vi "DAQ.DAQmx Replace Existing Task.vi"(9 "Task in":refnum<k21>, 10 "Task Index":i32, 11 "Tasks in":refnum<k21>[](array[refnum])) -> (3 "Tasks out":refnum<k21>[](array[refnum]))   [LabVIEW 2019, in "Instrument.Lockin.lvlib" / "Instrument.DAQ.lvclass"]
uses:
  Instrument.DAQ.lvclass
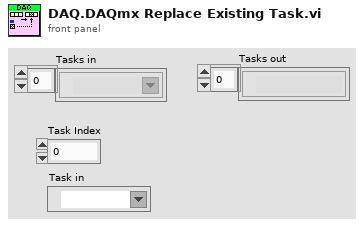
[diagram p1: front panel]
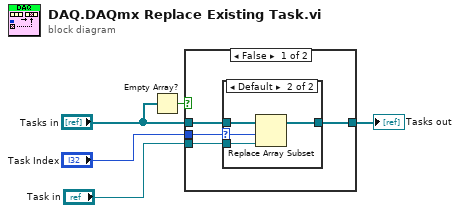
[diagram p0: block diagram]
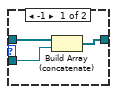
[diagram p2: hidden frame]
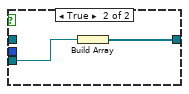
[diagram p3: hidden frame]
diagram:
  n1 = Empty Array?(array="Tasks in") -> (empty?=w1:bool)
  n2 = case shown="False" w1 {
    tunnel: [w9 w18] -> w3
    tunnel: "Task in" -> [w8 w17]
    tunnel: "Task Index" -> [w7 _]
    tunnel: "Tasks in" -> [w6 _]
    frame False {
      n3 = case shown="Default" w7 {
        selector: w7 -> [_ w14]
        tunnel: [w10 w16] -> w9
        tunnel: w8 -> [w11 w15]
        tunnel: w6 -> [w12 w13]
        frame -1 {
          n4 = Build Array (concatenate)(w12, w11) -> (w10:refnum<k21>[])
        }
        frame Default {
          n5 = Replace Array Subset(array=w13, new element=w15, index=w14) -> (w16:refnum<k21>[])
        }
      }
    }
    frame True {
      n6 = Build Array(w17) -> (w18:refnum<k21>[])
    }
  }
  "Tasks out" <- w3
